vi "U32BitSplit.vi"(1 "U32":u32 format="%032b") -> (0 "U8 Array":u8[](array[numeric]) format="%08b")   [LabVIEW 2014]
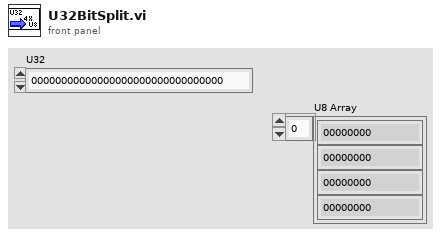
[diagram p1: front panel]
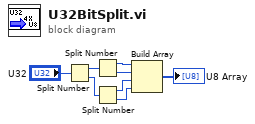
[diagram p0: block diagram]
diagram:
  n1 = Split Number(x="U32") -> (hi(x)=w7:u16, lo(x)=w6:u16)
  n2 = Split Number(x=w7) -> (hi(x)=w5:u8, lo(x)=w4:u8)
  n3 = Split Number(x=w6) -> (hi(x)=w3:u8, lo(x)=w2:u8)
  n4 = Build Array(w5, w4, w3, w2) -> (→"U8 Array":u8[])
